vi "Main.vi"() -> ()   [LabVIEW 2014]
doc: "Example of using standard HTTP protocol for recieving a web site (the HTML source)\n\n\nThis example uses the GET command. For general information about the HTTP protocol and other commands go to\nhttp://www.w3.org/Protocols\n\n\nBjornar Svingen\nbjornar.svingen@sintef.no bjornar.svingen@ktv.no"
panel:
  in  "drop frame backlog":bool
  out "# paths in queue":i32
  out "# images in queue":i32
  out "# packets in queue":i32
  out "Frame #":i32
  out "2D Picture":picture
  out "error out":errorcluster
  out "header":string
  out "Initial server response":string
  in  "stop":bool
  in  "remote port":u16=80
  in  "password":string
  in  "username":string="kirsch"
  in  "Camera address":string="10.0.7.103"
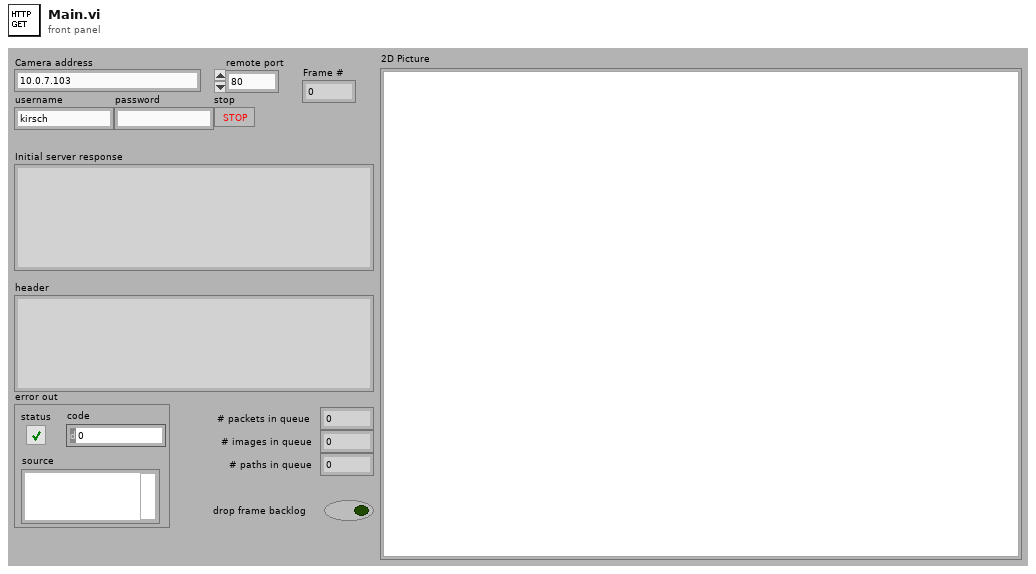
[diagram p1: front panel]
types:
  T1 = typedef "imagedata.ctl" = cluster{"image type":i32, "image depth":i32, "image":u8[], "mask":u8[], "colors":u32[], "Rectangle":cluster{"left":i16, "top":i16, "right":i16, "bottom":i16}}
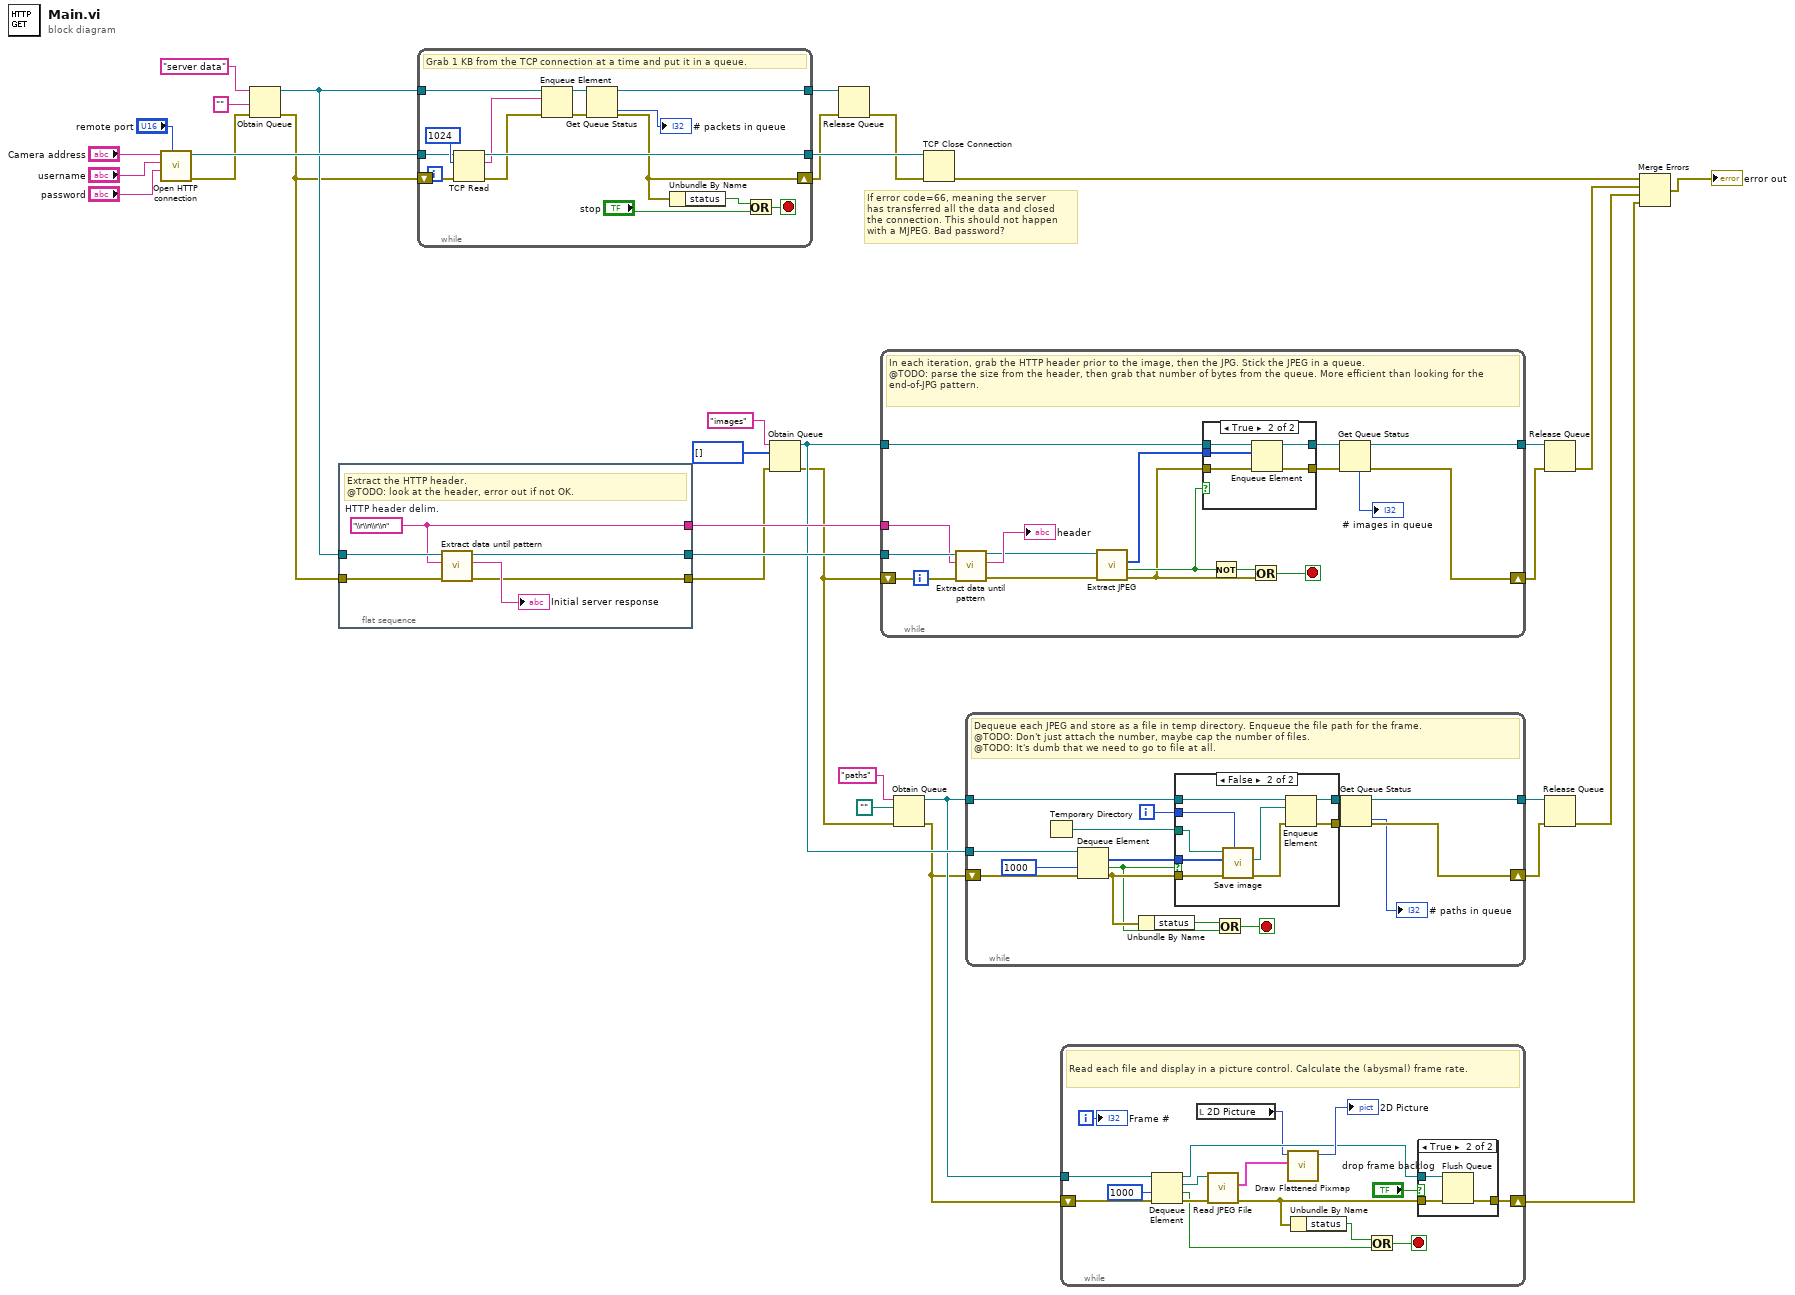
[diagram p0: block diagram]
diagram:
  # "If error code=66, meaning the server\nhas transferred all the data and closed\nthe connection. This should not happen\nwith a MJPEG. Bad password?"
  n1 = call "Open HTTP connection.vi"("remote port"="remote port", "password"="password", "username"="username", "Camera address"="Camera address") -> ("error out"=w10:errorcluster, "TCP Network Connection out"=w30:refnum<k5>)  [unwired: 6 in]
  n2 = Obtain Queue(name (unnamed)="server data", element data type="" ("name (unnamed)"), error in (no error)=w10) -> (queue out=w27:refnum<queue>, error out=w4:errorcluster)  [unwired: 2 in, 1 out]
  n3 = flat-sequence {
    tunnel: w27 -> [w40]
    tunnel: [w38] -> w26
    tunnel: w4 -> [w37]
    tunnel: [w36] -> w25
    tunnel: [w35] -> w3
    frame #0 {
      w36 = "\\r\\n\\r\\n"  # HTTP header delim.
      # "Extract the HTTP header.\n@TODO: look at the header, error out if not OK."
      n4 = call "Extract data until pattern.vi"("error in (no error)"=w37, "pattern to match"=w36, "Queue in"=w40) -> ("error out"=w35:errorcluster, "Data until pattern (inclusive)"=→"Initial server response":string, "Queue out"=w38:refnum<queue>)  [unwired: 6 in]
    }
  }
  n5 = while {
    tunnel: [w54] -> w18
    tunnel: w30 -> [w52]
    tunnel: w27 -> [w51]
    shift-right: [w42] -> w12
    shift-left: w4 -> [w55]
    tunnel: [w44] -> w24
    stop <- w49 stop-if-true
    # "Grab 1 KB from the TCP connection at a time and put it in a queue."
    n6 = TCP Read(connection ID=w52, bytes to read=1024, error in (no error)=w55) -> (connection ID out=w54:refnum<k5>, data out=w50:string, error out=w46:errorcluster)  [unwired: 2 in]
    n7 = Enqueue Element(queue=w51, element=w50, error in (no error)=w46) -> (queue out=w45:refnum<queue>, error out=w43:errorcluster)  [unwired: 1 in, 1 out]
    n8 = Get Queue Status(queue=w45, error in (no error)=w43) -> (queue out=w44:refnum<queue>, error out=w42:errorcluster, # elements in queue=→"# packets in queue":i32)  [unwired: 1 in, 5 out]
    n9 = Unbundle By Name(w42) -> ("status"=w48:bool)
    n10 = Or(x=w48, y="stop") -> (x .or. y?=w49:bool)
  }
  n11 = Obtain Queue(name (unnamed)="images", element data type=u8[] [] ("image data"), error in (no error)=w3) -> (queue out=w15:refnum<queue>, error out=w2:errorcluster)  [unwired: 2 in, 1 out]
  n12 = Release Queue(queue=w24, error in (no error)=w12) -> (error out=w11:errorcluster)  [unwired: 1 in, 2 out]
  n13 = while {
    tunnel: w26 -> [w72]
    tunnel: w25 -> [w69]
    shift-right: [w60] -> w7
    shift-left: w2 -> [w71]
    tunnel: w15 -> [w66]
    tunnel: [w62] -> w23
    stop <- w58 stop-if-true
    # "In each iteration, grab the HTTP header prior to the image, then the JPG. Stick the JPEG in a queue.\n@TODO: parse the size from the header, then grab that number of bytes from the queue. More efficient than looking for the end-of-JPG pattern."
    n14 = call "Extract data until pattern.vi"("error in (no error)"=w71, "pattern to match"=w69, "Queue in"=w72) -> ("error out"=w67:errorcluster, "Data until pattern (inclusive)"=→"header":string, "Queue out"=w68:refnum<queue>)  [unwired: 6 in]
    n15 = call "Extract JPEG.vi"("error in (no error)"=w67, "Queue in"=w68) -> ("error out"=w56:errorcluster, "valid image"=w64:bool, "image data"=w65:u8[])  [unwired: 6 in, 1 out]
    n16 = case shown="True" w64 {
      tunnel: w66 -> [w73 w79]
      tunnel: w56 -> [w74 w78]
      tunnel: w65 -> [_ w77]
      tunnel: [w74 w76] -> w61
      tunnel: [w73 w75] -> w63
      frame False {
      }
      frame True {
        n17 = Enqueue Element(queue=w79, element=w77, error in (no error)=w78) -> (queue out=w75:refnum<queue>, error out=w76:errorcluster)  [unwired: 1 in, 1 out]
      }
    }
    n18 = Not(x=w64) -> (.not. x?=w57:bool)
    n19 = Or(x=w57, y=w56) -> (x .or. y?=w58:bool)
    n20 = Get Queue Status(queue=w63, error in (no error)=w61) -> (queue out=w62:refnum<queue>, error out=w60:errorcluster, # elements in queue=→"# images in queue":i32)  [unwired: 1 in, 5 out]
  }
  n21 = Obtain Queue(name (unnamed)="paths", element data type=path "", error in (no error)=w2) -> (queue out=w14:refnum<queue>, error out=w1:errorcluster)  [unwired: 2 in, 1 out]
  n22 = TCP Close Connection(connection ID=w18, error in (no error)=w11) -> (error out=w13:errorcluster)  [unwired: 1 in, 1 out]
  n23 = while {
    shift-right: [w84] -> w9
    shift-left: w1 -> [w95]
    tunnel: w15 -> [w93]
    tunnel: w14 -> [w90]
    tunnel: [w82] -> w20
    i -> [w92]
    stop <- w87 stop-if-true
    # "Dequeue each JPEG and store as a file in temp directory. Enqueue the file path for the frame.\n@TODO: Don't just attach the number, maybe cap the number of files.\n@TODO: It's dumb that we need to go to file at all."
    n24 = Temporary Directory() -> (w80:path)
    n25 = Dequeue Element(queue=w93, timeout in ms (-1)=1000, error in (no error)=w95) -> (element=w91:u8[], timed out?=w86:bool, error out=w88:errorcluster)  [unwired: 1 out]
    n26 = Unbundle By Name(w88) -> ("status"=w89:bool)
    n27 = case shown="False" w86 {
      tunnel: w88 -> [w97 w106]
      tunnel: [w97 w98] -> w85
      tunnel: w80 -> [_ w105]
      tunnel: w92 -> [_ w104]
      tunnel: w91 -> [_ w103]
      tunnel: w90 -> [w96 w101]
      tunnel: [w96 w99] -> w83
      frame True {
      }
      frame False {
        n28 = call "Save image.vi"("image number"=w104, "error in"=w106, "image data"=w103, "folder (dialog)"=w105) -> ("error out"=w102:errorcluster, "image path"=w100:path)  [unwired: 6 in]
        n29 = Enqueue Element(queue=w101, element=w100, error in (no error)=w102) -> (queue out=w99:refnum<queue>, error out=w98:errorcluster)  [unwired: 1 in, 1 out]
      }
    }
    n30 = Or(x=w89, y=w86) -> (x .or. y?=w87:bool)
    n31 = Get Queue Status(queue=w83, error in (no error)=w85) -> (queue out=w82:refnum<queue>, error out=w84:errorcluster, # elements in queue=→"# paths in queue":i32)  [unwired: 1 in, 5 out]
  }
  n32 = while {
    tunnel: w14 -> [w122]
    shift-right: [w111] -> w19
    shift-left: w1 -> [w107]
    i -> [w116]
    stop <- w113 stop-if-true
    # "Read each file and display in a picture control. Calculate the (abysmal) frame rate."
    n33 = Dequeue Element(queue=w122, timeout in ms (-1)=1000, error in (no error)=w107) -> (queue out=w110:refnum<queue>, element=w119:path, timed out?=w114:bool, error out=w120:errorcluster)
    n34 = local read "2D Picture"() -> (w108:picture)
    n35 = call <vilib>:"Read JPEG File.vi"("error in (no error)"=w120, "path to JPEG file"=w119) -> ("error out"=w112:errorcluster, "image data"=w118:T1)  [unwired: 7 in, 1 out]
    n36 = call <vilib>:"Draw Flattened Pixmap.vi"("image data"=w118, "picture"=w108) -> ("new picture"=→"2D Picture":picture)  [unwired: 7 in]
    n37 = Unbundle By Name(w112) -> ("status"=w115:bool)
    n38 = Or(x=w115, y=w114) -> (x .or. y?=w113:bool)
    n39 = case shown="True" "drop frame backlog" {
      tunnel: w112 -> [w123 w126]
      tunnel: [w123 w125] -> w111
      tunnel: w110 -> [_ w124]
      frame False {
      }
      frame True {
        n40 = Flush Queue(queue=w124, error in (no error)=w126) -> (error out=w125:errorcluster)  [unwired: 2 out]
      }
    }
    "Frame #" <- w116
  }
  n41 = Release Queue(queue=w23, error in (no error)=w7) -> (error out=w6:errorcluster)  [unwired: 1 in, 2 out]
  n42 = Release Queue(queue=w20, error in (no error)=w9) -> (error out=w8:errorcluster)  [unwired: 1 in, 2 out]
  n43 = Merge Errors(w13, w6, w8, w19) -> (→"error out":errorcluster)
